vi "Keythley_2110.vi"(4 "error in":T14, 7 "Command":T15) -> (0 "error out":T14, 3 "Response":T12)   [LabVIEW 2018]
uses:
  MOKO_LabViewLibrary/MokoLowLevel/MokoLowLovelControl/MLLC_Command.ctl
  MOKO_LabViewLibrary/MokoLowLevel/MokoLowLovelControl/MLLC_Error.ctl
  MOKO_LabViewLibrary/MokoLowLevel/MokoLowLovelControl/MLLC_Mode.ctl
  MOKO_LabViewLibrary/MokoLowLevel/MokoLowLovelControl/MLLC_Response.ctl
  MOKO_LabViewLibrary/MokoLowLevel/MokoLowLovelControl/MLLC_DriverName.ctl
  MOKO_LabViewLibrary/MokoLowLevel/MokoLowLovelControl/MLLC_Request.ctl
  MOKO_LabViewLibrary/MokoLowLevel/MokoLowLovelControl/MLLC_ErrorCode.ctl
  MOKO_LabViewLibrary/MokoLowLevel/MokoLowLovelControl/MLLC_ResponseInit.ctl
  MOKO_LabViewLibrary/MokoLowLevel/MokoLowLovelControl/MLLC_ConnectCluster.ctl
  MOKO_LabViewLibrary/MokoLowLevel/MokoLowLovelControl/MLLC_InterfaceType.ctl
  MOKO_LabViewLibrary/MokoLowLevel/MokoLowLovelControl/MLLC_OpenedSession.ctl
  MOKO_LabViewLibrary/MokoLowLevel/MokoLowLovelControl/MLLC_InterfaceSettings.ctl
  MOKO_LabViewLibrary/MokoLowLevel/MokoLowLovelControl/MLLC_InterfaceKind.ctl
  data/Keythley_2110_Functions.ctl
panel:
  in  "Settings":T8={"Saved Data"=variant, "Data"={"Connect"={"InterfaceType"=enum."VISA", "OpenedSession"="USB0::0x05E6::0x2110::8000035::INSTR", "InterfaceSettings"={"Interface"=enum."USB", "EOS 4 read"=enum."LF (\\n)", "EOS 4 write"=enum."LF (\\n)", "TMO, ms"=5000, "Sett"=variant}}, "Channel"=1, "Func"=enum."VDC"}}
  in  "Response Init array":T9="KEITHLEY INSTRUMENTS INC.,MODEL 2110"
  in  "Error Code":T6=5475
  in  "Request":T10="*idn?"
  in  "Driver Name":T11="Keythley_2110"
  in  "Mode":T13=enum."Check"
  # "KEITHLEY INSTRUMENTS,MODEL DMM6500,04582450,1.7.12b = U"
  # "KEITHLEY INSTRUMENTS,MODEL DMM6500,04625545,1.7.12b = I"
  # "Keythley_2110"
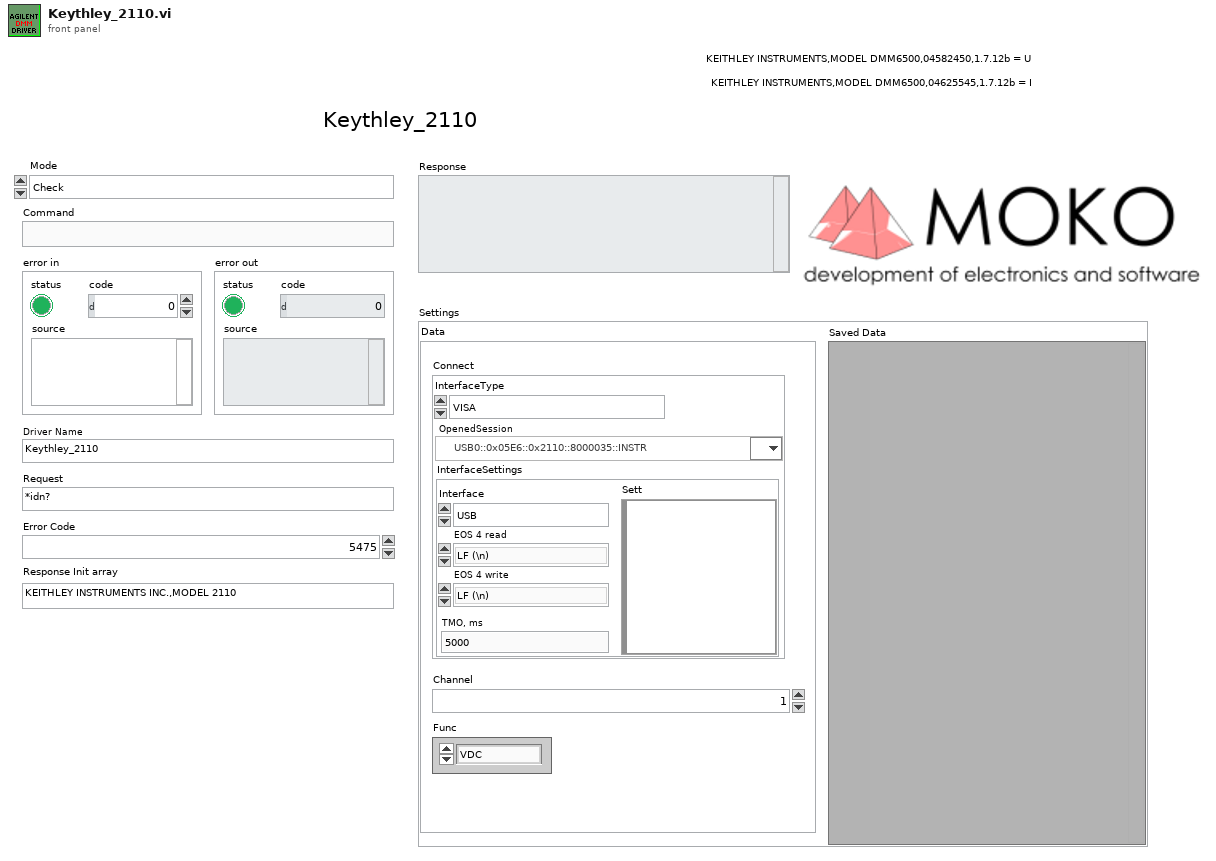
[diagram p1: front panel]
types:
  T1 = typedef "MLLC_ConnectCluster.ctl" = cluster{"InterfaceType":T2, "OpenedSession":T3, "InterfaceSettings":T4}
  T2 = typedef "MLLC_InterfaceType.ctl" = enum16{"VISA", "Prologix USB-GPIB"}
  T3 = typedef "MLLC_OpenedSession.ctl" = refnum<visa-resource-name>
  T4 = typedef "MLLC_InterfaceSettings.ctl" = cluster{"Interface":T5, "EOS 4 read":enum16{"Default (=EOS 4 write)", "CR (\\r)", "LF (\\n)", "None"}, "EOS 4 write":enum16{"CR+LF (\\r\\n)", "CR (\\r)", "LF (\\n)", "None"}, "TMO, ms":i32, "Sett":variant}
  T5 = typedef "MLLC_InterfaceKind.ctl" = enum16{"RS232", "GPIB", "USB", "Ethernet", "another"}
  T6 = typedef "MLLC_ErrorCode.ctl" = u32
  T7 = typedef "Keythley_2110_Functions.ctl" = enum16{"VDC", "VAC", "IDC", "IAC", "F", "R2", "R4", "CAP"}
  T8 = cluster{"Saved Data":variant, "Data":cluster{"Connect":T1, "Channel":T6, "Func":T7}}
  T9 = typedef "MLLC_ResponseInit.ctl" = string
  T10 = typedef "MLLC_Request.ctl" = string
  T11 = typedef "MLLC_DriverName.ctl" = string
  T12 = typedef "MLLC_Response.ctl" = string
  T13 = typedef "MLLC_Mode.ctl" = enum16{"get", "set", "close", "Init", "Check"}
  T14 = typedef "MLLC_Error.ctl" = errorcluster
  T15 = typedef "MLLC_Command.ctl" = string
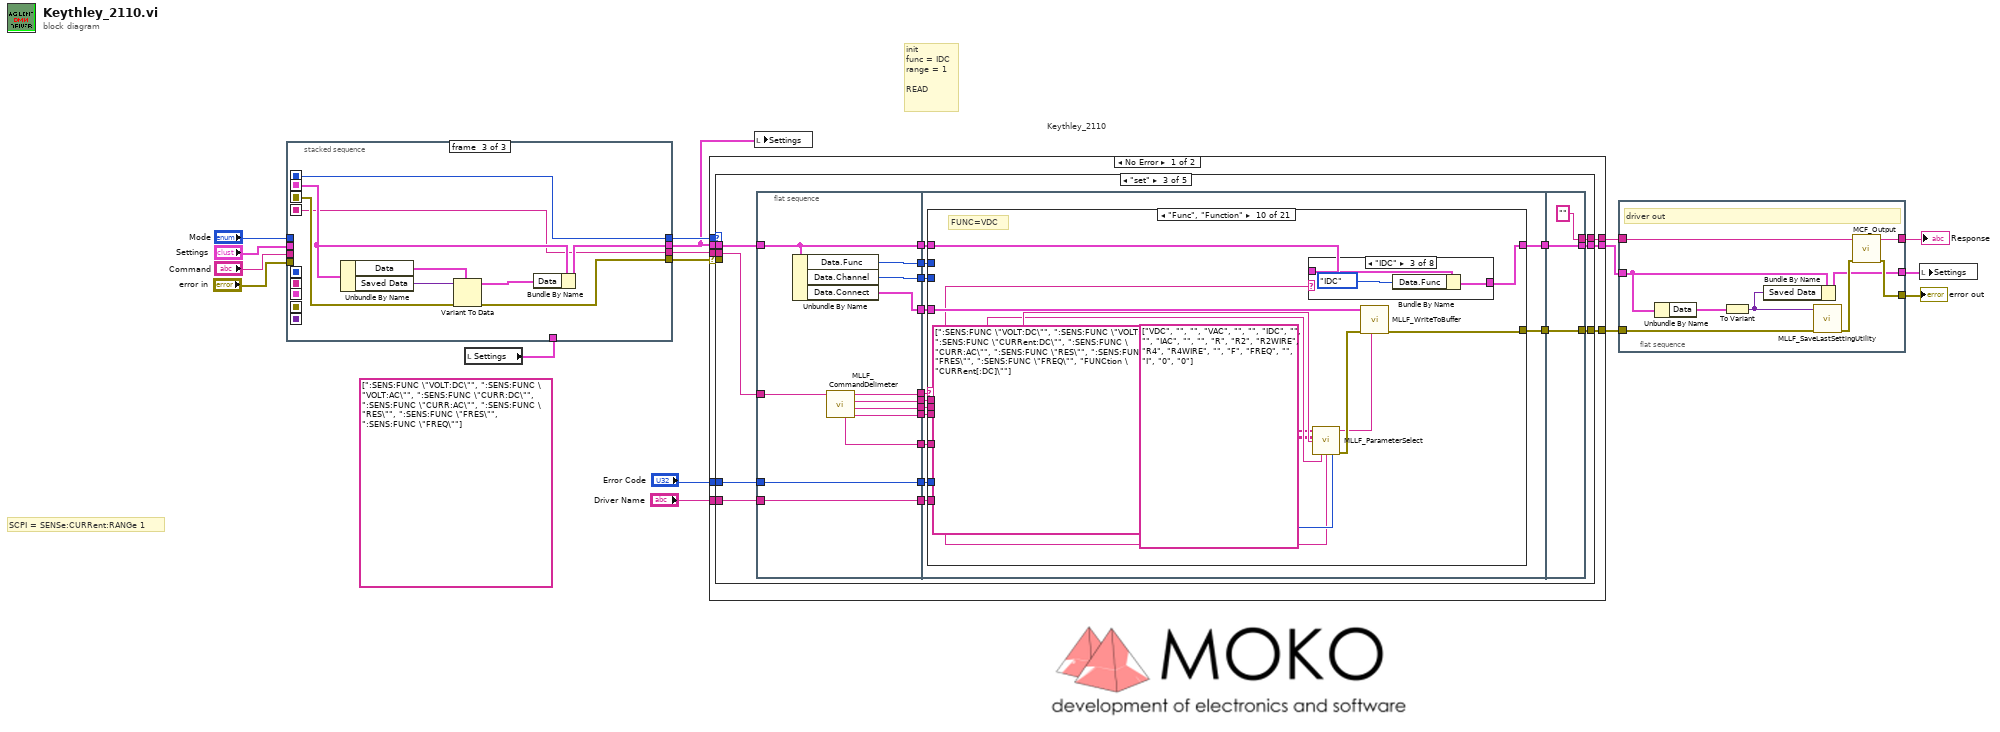
[diagram p0: block diagram]
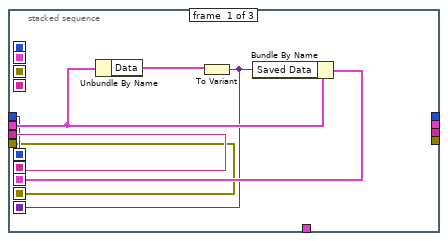
[diagram p2: hidden frame]
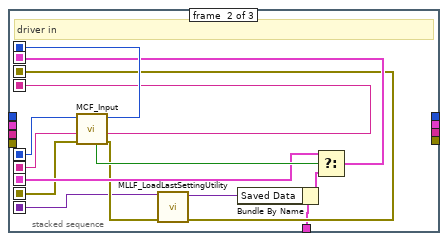
[diagram p3: hidden frame]
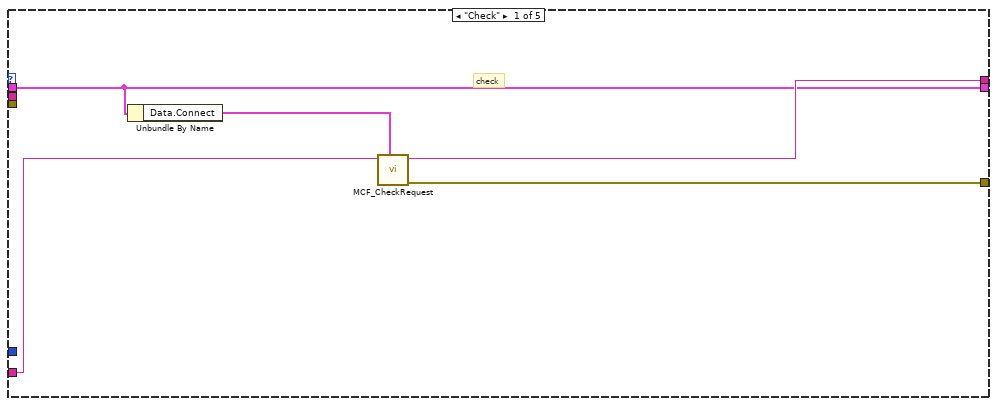
[diagram p4: hidden frame]
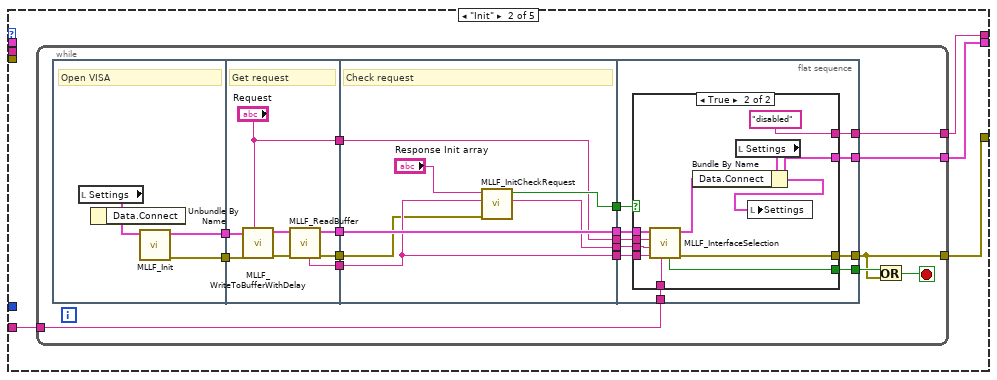
[diagram p5: hidden frame]
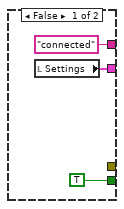
[diagram p6: hidden frame]
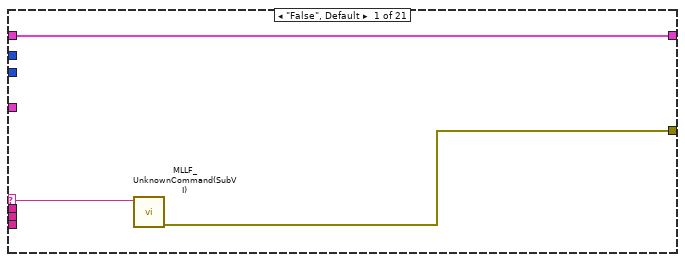
[diagram p7: hidden frame]
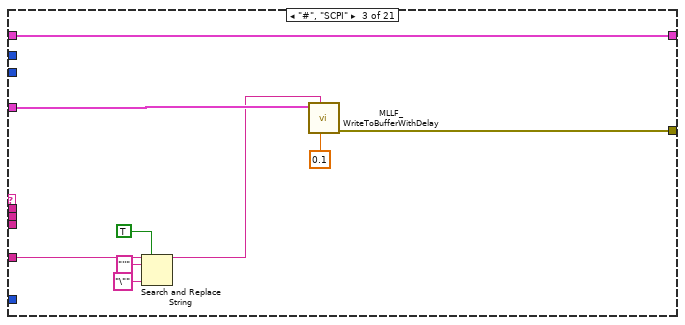
[diagram p9: hidden frame]
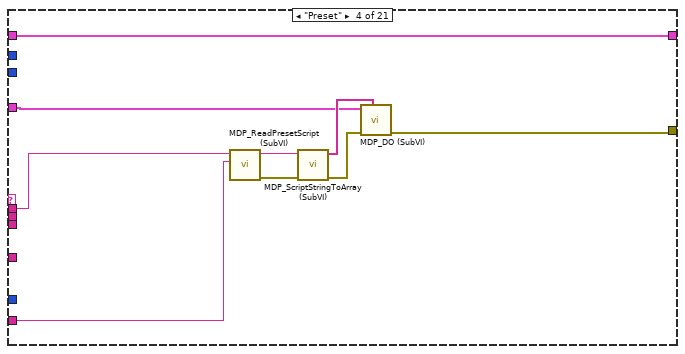
[diagram p10: hidden frame]
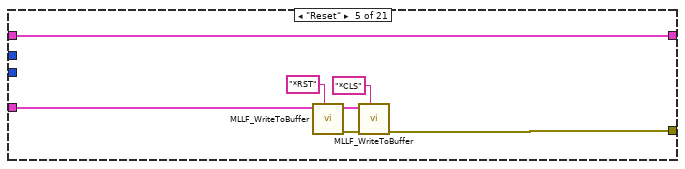
[diagram p11: hidden frame]
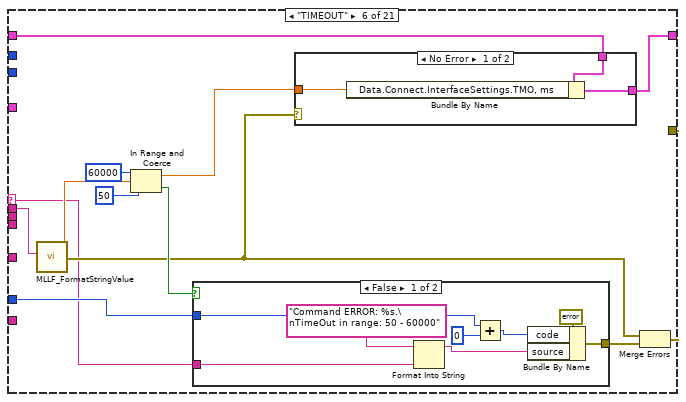
[diagram p12: hidden frame]
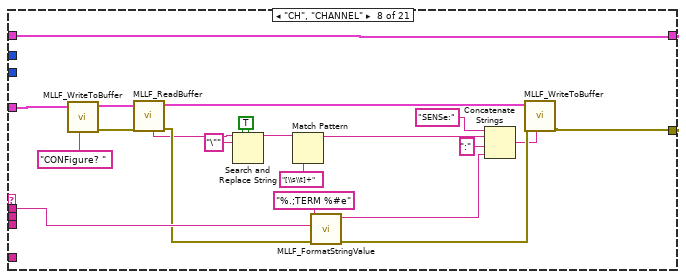
[diagram p16: hidden frame]
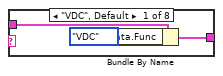
[diagram p18: hidden frame]
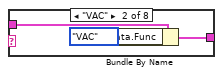
[diagram p19: hidden frame]
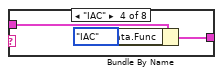
[diagram p20: hidden frame]
diagram:
  (unwired) string[] [":SENS:FUNC \"VOLT:DC\"", ":SENS:FUNC \"VOLT:AC\"", ":SENS:FUNC \"CURR:DC\"", ":SENS:FUNC \"CURR:AC\"", ":SENS:FUNC \"RES\"", ":SENS:FUNC \"FRES\"", ":SENS:FUNC \"FREQ\""] ("Names")
  # "init\nfunc = IDC\nrange = 1\n\nREAD"
  # "SCPI = SENSe:CURRent:RANGe 1"
  # "Keythley_2110"
  n1 = local read "Settings"() -> (w8:T8)
  n2 = stacked-sequence {
    seq-local: [w20 _ _] -> [_ w36 _]
    seq-local: [w19 _ _] -> [_ w37 _]
    seq-local: [w22 _ _] -> [_ w32 _]
    seq-local: [w18 _ _] -> [_ w31 _]
    seq-local: [w21 _ _] -> [_ w27 _]
    seq-local: [_ w28 _] -> [_ _ w44]
    seq-local: [_ w38 _] -> [_ _ w41]
    seq-local: [_ w35 _] -> [_ _ w40]
    seq-local: [_ w34 _] -> [_ _ w45]
    tunnel: "Command" -> [w20 _ _]
    tunnel: "Mode" -> [w19 _ _]
    tunnel: "error in" -> [w18 _ _]
    tunnel: "Settings" -> [w23 _ _]
    tunnel: w8 -> [_ w26 _]
    tunnel: [_ _ w40] -> w10
    tunnel: [_ _ w43] -> w1
    tunnel: [_ _ w42] -> w9
    tunnel: [_ _ w41] -> w11
    frame #0 {
      n3 = Unbundle By Name(w23) -> ("Data"=w24:cluster{"Connect":T1, "Channel":T6, "Func":T7})
      n4 = To Variant(anything=w24) -> (Variant=w21:variant)
      n5 = Bundle By Name(cluster=w23, "Saved Data"=w21) -> (w22:T8)
    }
    frame #1 {
      # "driver in"
      n6 = call "MCF_Input.vi"("Error In"=w31, "Command in"=w36, "Mode in"=w37) -> ("Error Out"=w30:errorcluster, "Command out"=w35:string, "Mode out"=w38:T13, "Boolean"=w33:bool)  [unwired: 5 in]
      n7 = call "MLLF_LoadLastSettingUtility.vi"("Error In"=w30, "Save data in"=w27) -> ("Error Out"=w28:errorcluster, "Save data out"=w25:variant)  [unwired: 8 in]
      n8 = Bundle By Name(cluster=w26, "Saved Data"=w25) -> (w29:T8)
      n9 = Select(t=w32, s=w33, f=w29) -> (s? t:f=w34:T8)
    }
    frame #2 {
      n10 = Unbundle By Name(w45) -> ("Data"=w46:cluster{"Connect":T1, "Channel":T6, "Func":T7}, "Saved Data"=w39:variant)
      n11 = Variant To Data(error in=w44, type=w46, Variant=w39) -> (data=w47:cluster{"Connect":T1, "Channel":T6, "Func":T7}, error out=w42:errorcluster)
      n12 = Bundle By Name(cluster=w45, "Data"=w47) -> (w43:T8)
    }
  }
  n13 = case shown="No Error" w9 {
    selector: w9 -> [w53 w615]
    tunnel: [w54 w615] -> w5
    tunnel: w11 -> [w56 _]
    tunnel: [w55 "An error occurred in the driver input module." ("String")] -> w7
    tunnel: w10 -> [w48 _]
    tunnel: w1 -> [w49 w614]
    tunnel: "Error Code" -> [w52 _]
    tunnel: "Driver Name" -> [w51 _]
    tunnel: [w50 w614] -> w6
    frame No Error {
      n14 = case shown="\"set\"" w56 {
        tunnel: [w60 w65 w139 w524 "" ("String")] -> w55
        tunnel: [w61 w63 w142 w525 w611] -> w54
        tunnel: w53 -> [_ _ _ w539 _]
        tunnel: w52 -> [_ _ w145 w541 _]
        tunnel: w51 -> [w59 w62 w143 w540 _]
        tunnel: [w58 w64 w144 w542 w610] -> w50
        tunnel: w49 -> [w58 _ w128 w530 w610]
        tunnel: w48 -> [_ _ w127 w529 _]
        frame "Check" {
          # "check"
          n15 = Unbundle By Name(w58) -> ("Data.Connect"=w57:T1)
          n16 = call "MCF_CheckRequest.vi"("Permanent data.Connect"=w57, "Driver Name"=w59) -> ("Error Out"=w61:errorcluster, "Output String"=w60:string)  [unwired: 8 in]
        }
        frame "Init" {
          n17 = while {
            tunnel: [w71] -> w63
            tunnel: [w70] -> w65
            tunnel: [w69] -> w64
            tunnel: w62 -> [w73]
            stop <- w82 stop-if-true
            n18 = flat-sequence {
              tunnel: [w86] -> w81
              tunnel: [w85] -> w80
              tunnel: w81 -> [w92]
              tunnel: w80 -> [w91]
              tunnel: [w90] -> w79
              tunnel: [w89] -> w78
              tunnel: [w88] -> w77
              tunnel: ["Request"] -> w67
              tunnel: w79 -> [w98]
              tunnel: w78 -> [w101]
              tunnel: w77 -> [w100]
              tunnel: [w101] -> w76
              tunnel: [w100] -> w75
              tunnel: [w97] -> w74
              tunnel: [w96] -> w68
              tunnel: w67 -> [w95]
              tunnel: [w95] -> w66
              tunnel: w76 -> [w110]
              tunnel: w75 -> [w109]
              tunnel: w74 -> [w111]
              tunnel: w73 -> [w108]
              tunnel: [w107] -> w72
              tunnel: [w106] -> w71
              tunnel: [w105] -> w70
              tunnel: [w104] -> w69
              tunnel: w68 -> [w103]
              tunnel: w66 -> [w102]
              frame #0 {
                # "Open VISA"
                n19 = local read "Settings"() -> (w84:T8)
                n20 = Unbundle By Name(w84) -> ("Data.Connect"=w83:T1)
                n21 = call "MLLF_Init.vi"("DriverConnect in"=w83) -> ("Error Out"=w86:errorcluster, "DriverConnect out"=w85:T1)  [unwired: 7 in]
              }
              frame #1 {
                # "Get request"
                n22 = call "MLLF_WriteToBufferWithDelay.vi"("Command"="Request", "Error In"=w92, "DriverConnect in"=w91) -> ("Error Out"=w93:errorcluster, "DriverConnect out"=w94:T1)  [unwired: 7 in]
                n23 = call "MLLF_ReadBuffer.vi"("Error In"=w93, "DriverConnect in"=w94) -> ("Error Out"=w90:errorcluster, "DriverConnect out"=w89:T1, "String"=w88:string)  [unwired: 6 in]
              }
              frame #2 {
                # "Check request"
                n24 = call "MLLF_InitCheckRequest.vi"("error in (no error)"=w98, "Answer"=w100, "Response Init"="Response Init array") -> ("ResponseInit out"=w96:string, "Design"=w97:bool)  [unwired: 5 in, 2 out]
              }
              frame #3 {
                n25 = case shown="True" w111 {
                  tunnel: w110 -> [_ w124]
                  tunnel: [TRUE w119] -> w107
                  tunnel: [_ w122] -> w106
                  tunnel: ["connected" "disabled"] -> w105
                  tunnel: [w112 w120] -> w104
                  tunnel: w109 -> [_ w117]
                  tunnel: w108 -> [_ w118]
                  tunnel: w103 -> [_ w116]
                  tunnel: w102 -> [_ w115]
                  frame False {
                    n26 = local read "Settings"() -> (w112:T8)
                  }
                  frame True {
                    n27 = call "MLLF_InterfaceSelection.vi"("Driver Name"=w118, "Answer:"=w117, "Response"=w116, "Request"=w115, "DriverConnect in"=w124) -> ("error out"=w122:T14, "DriverConnect out"=w123:T1, "stop init?"=w119:bool)  [unwired: 2 in, 2 out]
                    n28 = local read "Settings"() -> (w125:T8)
                    n29 = Bundle By Name(cluster=w125, "Data.Connect"=w123) -> (w120:T8)
                    n30 = local write "Settings"(w120) -> ()
                  }
                }
              }
            }
            n31 = Or(x=w72, y=w71) -> (x .or. y?=w82:bool)
          }
        }
        frame "set" {
          n32 = flat-sequence {
            tunnel: w143 -> [w156]
            tunnel: w128 -> [w147]
            tunnel: w145 -> [w157]
            tunnel: [w157] -> w138
            tunnel: [w147] -> w137
            tunnel: [w156] -> w136
            tunnel: [w153] -> w135
            tunnel: [w154] -> w134
            tunnel: [w155] -> w133
            tunnel: [w148] -> w132
            tunnel: [w149] -> w131
            tunnel: [w150] -> w130
            tunnel: [w151] -> w129
            tunnel: w127 -> [w152]
            tunnel: [w146] -> w126
            tunnel: [w168] -> w141
            tunnel: [w161] -> w140
            tunnel: w138 -> [w170]
            tunnel: w137 -> [w169]
            tunnel: w136 -> [w167]
            tunnel: w135 -> [w166]
            tunnel: w134 -> [w165]
            tunnel: w133 -> [w164]
            tunnel: w132 -> [w163]
            tunnel: w131 -> [w162]
            tunnel: w130 -> [w160]
            tunnel: w129 -> [w159]
            tunnel: w126 -> [w158]
            tunnel: [w522] -> w142
            tunnel: [w523] -> w144
            tunnel: w141 -> [w523]
            tunnel: w140 -> [w522]
            tunnel: ["" ("String")] -> w139
            frame #0 {
              n33 = Unbundle By Name(w147) -> ("Data.Func"=w155:T7, "Data.Channel"=w154:T6, "Data.Connect"=w153:T1)
              n34 = call "MLLF_CommandDelimeter.vi"("command with param"=w152) -> ("param 3"=w151:string, "param 2"=w150:string, "param 1"=w149:string, "command"=w148:string, "Spit delimetre"=w146:string)  [unwired: 6 in]
            }
            frame #1 {
              n35 = case shown="\"Func\", \"Function\"" w163 {
                selector: w163 -> [w172 _ _ _ _ w201 _ _ _ w253 _ _ _ _ _ _ w445 w452 w476 w500 w511]
                tunnel: w162 -> [_ _ _ w187 _ w200 _ w244 _ w254 w293 _ w323 w336 w377 w407 w446 w453 w477 w501 w512]
                tunnel: [w171 _ w180 w184 w193 w206 _ w226 _ w248 w288 _ w306 w335 w361 w392 w425 w451 w475 w499 w510] -> w161
                tunnel: w170 -> [_ _ _ _ _ w207 _ _ _ w259 _ _ _ _ _ _ w447 w457 w481 w505 w519]
                tunnel: w169 -> [w173 w174 w183 w192 w199 w211 w225 w245 w247 w256 w294 w305 w325 w352 w379 w409 w450 w474 w498 w509 w520]
                tunnel: [w173 w174 w183 w192 w199 w212 w225 w245 w247 w255 w294 w305 w325 w352 w379 w409 w450 w474 w498 w509 w520] -> w168
                tunnel: w166 -> [_ _ w181 w185 w194 _ _ w246 _ w257 w286 _ w324 w351 w378 w408 w449 w473 w497 w503 w516]
                tunnel: w167 -> [_ _ _ w186 _ _ _ _ _ w258 _ _ _ _ _ _ w448 w458 w482 w506 w518]
                tunnel: w165 -> [_ _ _ _ _ _ _ _ _ _ _ _ _ _ _ _ _ _ _ _ _]
                tunnel: w164 -> [_ _ _ _ _ _ _ _ _ _ w287 _ _ _ _ _ _ _ _ _ _]
                tunnel: w160 -> [_ _ _ _ _ _ _ _ _ _ _ _ _ _ _ _ _ _ _ _ _]
                tunnel: w159 -> [_ _ _ _ _ _ _ _ _ _ _ _ _ _ _ _ _ _ _ _ _]
                tunnel: w158 -> [_ _ w179 _ _ _ _ _ _ _ _ _ _ _ _ _ _ _ _ _ _]
                frame "False", Default {
                  n36 = call "MLLF_UnknownCommand(SubVI).vi"("Unknown command"=w172) -> ("error out"=w171:errorcluster)  [unwired: 10 in]
                }
                frame "______________ Standart ________________" {
                }
                frame "#", "SCPI" {
                  n37 = Search and Replace String(replace all?=TRUE ("replace all? (F)"), input string=w179, search string="''", replace string="\"" ("replace string (\"\")")) -> (result string=w175:string)  [unwired: 4 in, 3 out]
                  n38 = call "MLLF_WriteToBufferWithDelay.vi"("Delay Time ( 0,05 s)"=0.1 ("Delay Time (s)"), "Command"=w175, "DriverConnect in"=w181) -> ("Error Out"=w180:errorcluster)  [unwired: 7 in, 1 out]
                }
                frame "Preset" {
                  n39 = call "MDP_ReadPresetScript (SubVI).vi"("Driver Name"=w186, "String in"=w187) -> ("Error Out"=w189:errorcluster, "String out"=w190:string)  [unwired: 8 in]
                  n40 = call "MDP_ScriptStringToArray (SubVI).vi"("Error In"=w189, "String script"=w190) -> ("Error Out"=w191:errorcluster, "Array script"=w188:string[])  [unwired: 8 in]
                  n41 = call "MDP_DO (SubVI).vi"("Array script"=w188, "Error in (no error)"=w191, "DriverConnect in"=w185) -> ("Error Out"=w184:errorcluster)  [unwired: 7 in, 1 out]
                }
                frame "Reset" {
                  n42 = call "MLLF_WriteToBuffer.vi"("String"="*RST", "DriverConnect in"=w194) -> ("error out"=w197:T14, "DriverConnect out"=w198:T1)  [unwired: 6 in]
                  n43 = call "MLLF_WriteToBuffer.vi"("String"="*CLS" ("write buffer"), "error in"=w197, "DriverConnect in"=w198) -> ("error out"=w193:T14)  [unwired: 5 in, 1 out]
                }
                frame "TIMEOUT" {
                  n44 = call "MLLF_FormatStringValue.vi"("String Value"=w200) -> ("error out"=w202:T14, "number"=w203:dbl)  [unwired: 8 in, 1 out]
                  n45 = In Range and Coerce(upper limit=60000, x=w203, lower limit=50) -> (coerced(x)=w208:dbl, In Range?=w204:bool)
                  n46 = case shown="False" w204 {
                    tunnel: [w219 _] -> w205
                    tunnel: w207 -> [w218 _]
                    tunnel: w201 -> [w217 _]
                    frame False {
                      n47 = Format Into String(format string="Command ERROR: %s.\nTimeOut in range: 50 - 60000", w217) -> (resulting string=w221:string)  [unwired: 2 in, 1 out]
                      n48 = Add(x=w218, y=0) -> (x+y=w222:T6)
                      n49 = Bundle By Name(cluster=errorcluster {"status"=TRUE, "code"=0, "source"=""} ("error out"), "code"=w222, "source"=w221) -> (w219:errorcluster)
                    }
                    frame True {
                    }
                  }
                  n50 = case shown="No Error" w202 {
                    tunnel: [w215 w216] -> w212
                    tunnel: w211 -> [w214 w216]
                    tunnel: w208 -> [w213 _]
                    frame No Error {
                      n51 = Bundle By Name(cluster=w214, "Data.Connect.InterfaceSettings.TMO, ms"=w213) -> (w215:T8)
                    }
                    frame Error {
                    }
                  }
                  n52 = Merge Errors(w202, w205) -> (w206:errorcluster)
                }
                frame "________________________________________" {
                }
                frame "CH", "CHANNEL" {
                  w231 = TRUE ("replace all? (F)")
                  n53 = call "MLLF_WriteToBuffer.vi"("String"="CONFigure? ", "DriverConnect in"=w246) -> ("error out"=w240:T14, "DriverConnect out"=w241:T1)  [unwired: 6 in]
                  n54 = call "MLLF_ReadBuffer.vi"("Error In"=w240, "DriverConnect in"=w241) -> ("Error Out"=w239:errorcluster, "DriverConnect out"=w238:T1, "String"=w233:string)  [unwired: 6 in]
                  n55 = Search and Replace String(replace all?=w231, case sensitive?=w231, input string=w233, search string="\"") -> (result string=w232:string)  [unwired: 4 in, 3 out]
                  n56 = Match Pattern(string=w232, regular expression="[\\s\\t]+") -> (before substring=w234:string)  [unwired: 1 in, 3 out]
                  n57 = call "MLLF_FormatStringValue.vi"("error in"=w239, "String Value"=w244, "Format"="%.;TERM %#e" ("format string")) -> ("error out"=w243:T14, "String Value Formated"=w236:T15)  [unwired: 6 in, 1 out]
                  n58 = Concatenate Strings("SENSe:" ("string"), w234, ":" ("string"), w236) -> (w229:string)
                  n59 = call "MLLF_WriteToBuffer.vi"("String"=w229, "error in"=w243, "DriverConnect in"=w238) -> ("error out"=w226:T14)  [unwired: 5 in, 1 out]
                }
                frame "<----MAIN FUNCTIONS---->" {
                }
                frame "Func", "Function" {
                  # "FUNC=VDC"
                  n60 = case shown="\"IDC\"" w254 {
                    tunnel: w256 -> [w262 w265 w268 w271 w274 w277 w280 w283]
                    tunnel: [w261 w264 w267 w270 w273 w276 w279 w282] -> w255
                    frame "VDC", Default {
                      n61 = Bundle By Name(cluster=w262, "Data.Func"=Keythley_2110_Functions."VDC" ("Func")) -> (w261:T8)
                    }
                    frame "VAC" {
                      n62 = Bundle By Name(cluster=w265, "Data.Func"=Keythley_2110_Functions."VAC" ("Func")) -> (w264:T8)
                    }
                    frame "IDC" {
                      n63 = Bundle By Name(cluster=w268, "Data.Func"=Keythley_2110_Functions."IDC" ("Func")) -> (w267:T8)
                    }
                    frame "IAC" {
                      n64 = Bundle By Name(cluster=w271, "Data.Func"=Keythley_2110_Functions."IAC" ("Func")) -> (w270:T8)
                    }
                    frame "R", "R2", "R2WI" {
                      n65 = Bundle By Name(cluster=w274, "Data.Func"=Keythley_2110_Functions."R2" ("Func")) -> (w273:T8)
                    }
                    frame "R4", "R4WI" {
                      n66 = Bundle By Name(cluster=w277, "Data.Func"=Keythley_2110_Functions."R4" ("Func")) -> (w276:T8)
                    }
                    frame "F" {
                      n67 = Bundle By Name(cluster=w280, "Data.Func"=Keythley_2110_Functions."F" ("Func")) -> (w279:T8)
                    }
                    frame "C", "CAP" {
                      n68 = Bundle By Name(cluster=w283, "Data.Func"=Keythley_2110_Functions."CAP" ("Func")) -> (w282:T8)
                    }
                  }
                  n69 = call "MLLF_ParameterSelect.vi"("Command to equipment"=string[] [":SENS:FUNC \"VOLT:DC\"", ":SENS:FUNC \"VOLT:AC\"", ":SENS:FUNC \"CURRent:DC\"", ":SENS:FUNC \"CURR:AC\"", ":SENS:FUNC \"RES\"", ":SENS:FUNC \"FRES\"", ":SENS:FUNC \"FREQ\"", "FUNCtion \"CURRent[:DC]\""] ("Names"), "Names"=string[][] [["VDC", "", ""], ["VAC", "", ""], ["IDC", "", ""], ["IAC", "", ""], ["R", "R2", "R2WIRE"], ["R4", "R4WIRE", ""], ["F", "FREQ", ""], ["I", "0", "0"]], "Input"=w254, "Command"=w253, "Driver Name"=w258, "Error Code"=w259) -> ("Choice"=w249:string, "Error Out"=w250:errorcluster)  [unwired: 8 in]
                  n70 = call "MLLF_WriteToBuffer.vi"("String"=w249, "error in"=w250, "DriverConnect in"=w257) -> ("error out"=w248:T14)  [unwired: 5 in, 1 out]
                }
                frame "Range" {
                  n71 = case shown="\"IDC\"" w287 {
                    tunnel: ["VOLT" ("String") "VOLT:AC" ("String") "CURR:DC" ("String")] -> w285
                    frame "VDC", Default {
                    }
                    frame "VAC" {
                    }
                    frame "IDC" {
                    }
                  }
                  n72 = case shown="Default" w293 {
                    selector: w293 -> [w298 _ _ _]
                    tunnel: [w301 _ _ _] -> w292
                    tunnel: [w300 "RANG:AUTO ON" ("String") "RANG MIN" ("String") "RANG MAX" ("String")] -> w291
                    frame Default {
                      n73 = call "MLLF_FormatStringValue.vi"("String Value"=w298, "Format"="RANG %#e" ("format string")) -> ("error out"=w301:T14, "String Value Formated"=w300:T15)  [unwired: 7 in, 1 out]
                    }
                    frame "Auto" {
                    }
                    frame "MIN" {
                    }
                    frame "MAX" {
                    }
                  }
                  n74 = Concatenate Strings("SENSe:" ("string"), w285, ":" ("string"), w291) -> (w289:string)
                  n75 = call "MLLF_WriteToBuffer.vi"("String"=w289, "error in"=w292, "DriverConnect in"=w286) -> ("error out"=w288:T14)  [unwired: 5 in, 1 out]
                }
                frame "---------ADDITIONAL---------" {
                }
                frame "Res", "Resolution" {
                  w310 = TRUE ("replace all? (F)")
                  n76 = call "MLLF_WriteToBuffer.vi"("String"="CONFigure? ", "DriverConnect in"=w324) -> ("error out"=w319:T14, "DriverConnect out"=w320:T1)  [unwired: 6 in]
                  n77 = call "MLLF_ReadBuffer.vi"("Error In"=w319, "DriverConnect in"=w320) -> ("Error Out"=w318:errorcluster, "DriverConnect out"=w317:T1, "String"=w312:string)  [unwired: 6 in]
                  n78 = Search and Replace String(replace all?=w310, case sensitive?=w310, input string=w312, search string="\"") -> (result string=w311:string)  [unwired: 4 in, 3 out]
                  n79 = case shown="\"MIN\"" w323 {
                    selector: w323 -> [w327 _ _]
                    tunnel: [w330 w331 w333] -> w322
                    tunnel: [w329 "RES MAX" ("String") "RES MIN" ("String")] -> w315
                    tunnel: w318 -> [w326 w331 w333]
                    frame "False", Default {
                      n80 = call "MLLF_FormatStringValue.vi"("error in"=w326, "String Value"=w327, "Format"="RES %#e" ("format string")) -> ("error out"=w330:T14, "String Value Formated"=w329:T15)  [unwired: 6 in, 1 out]
                    }
                    frame "MAX" {
                    }
                    frame "MIN" {
                    }
                  }
                  n81 = Match Pattern(string=w311, regular expression="[\\s\\t]+") -> (before substring=w313:string)  [unwired: 1 in, 3 out]
                  n82 = Concatenate Strings("SENSe:" ("string"), w313, ":" ("string"), w315) -> (w308:string)
                  n83 = call "MLLF_WriteToBuffer.vi"("String"=w308, "error in"=w322, "DriverConnect in"=w317) -> ("error out"=w306:T14)  [unwired: 5 in, 1 out]
                }
                frame "Aper", "Aperture", "MeasTime" {
                  w339 = TRUE ("replace all? (F)")
                  n84 = call "MLLF_WriteToBuffer.vi"("String"="CONFigure? ", "DriverConnect in"=w351) -> ("error out"=w348:T14, "DriverConnect out"=w349:T1)  [unwired: 6 in]
                  n85 = call "MLLF_ReadBuffer.vi"("Error In"=w348, "DriverConnect in"=w349) -> ("Error Out"=w347:errorcluster, "DriverConnect out"=w346:T1, "String"=w341:string)  [unwired: 6 in]
                  n86 = Search and Replace String(replace all?=w339, case sensitive?=w339, input string=w341, search string="\"") -> (result string=w340:string)  [unwired: 4 in, 3 out]
                  n87 = case shown="\"OFF\"" w336 {
                    selector: w336 -> [w355 _]
                    tunnel: [w358 w359] -> w353
                    tunnel: [w357 "APER:ENAB OFF" ("String")] -> w344
                    tunnel: w347 -> [w354 w359]
                    frame "False", Default {
                      n88 = call "MLLF_FormatStringValue.vi"("error in"=w354, "String Value"=w355, "Format"="APER %#e" ("format string")) -> ("error out"=w358:T14, "String Value Formated"=w357:T15)  [unwired: 6 in, 1 out]
                    }
                    frame "OFF" {
                    }
                  }
                  n89 = Match Pattern(string=w340, regular expression="[\\s\\t]+") -> (before substring=w342:string)  [unwired: 1 in, 3 out]
                  n90 = Concatenate Strings(w342, ":" ("string"), w344) -> (w337:string)
                  n91 = call "MLLF_WriteToBuffer.vi"("String"=w337, "error in"=w353, "DriverConnect in"=w346) -> ("error out"=w335:T14)  [unwired: 5 in, 1 out]
                }
                frame "IntegrationTime", "IntTime", "NPLC" {
                  w365 = TRUE ("replace all? (F)")
                  n92 = call "MLLF_WriteToBuffer.vi"("String"="CONFigure? ", "DriverConnect in"=w378) -> ("error out"=w373:T14, "DriverConnect out"=w374:T1)  [unwired: 6 in]
                  n93 = call "MLLF_ReadBuffer.vi"("Error In"=w373, "DriverConnect in"=w374) -> ("DriverConnect out"=w372:T1, "String"=w367:string)  [unwired: 6 in, 1 out]
                  n94 = Search and Replace String(replace all?=w365, case sensitive?=w365, input string=w367, search string="\"") -> (result string=w366:string)  [unwired: 4 in, 3 out]
                  n95 = case shown="\"MIN\"" w377 {
                    tunnel: [w383 w387 w391] -> w376
                    tunnel: [w382 w386 w390] -> w370
                    tunnel: w377 -> [w380 w384 w388]
                    frame Default {
                      n96 = call "MLLF_FormatStringValue.vi"("String Value"=w380, "Format"="NPLC %#e" ("format string")) -> ("error out"=w383:T14, "String Value Formated"=w382:T15)  [unwired: 7 in, 1 out]
                    }
                    frame "MIN" {
                      n97 = call "MLLF_FormatStringValue.vi"("String Value"=w384, "Format"="NPLC MIN" ("format string")) -> ("error out"=w387:T14, "String Value Formated"=w386:T15)  [unwired: 7 in, 1 out]
                    }
                    frame "MAX" {
                      n98 = call "MLLF_FormatStringValue.vi"("String Value"=w388, "Format"="NPLC MAX" ("format string")) -> ("error out"=w391:T14, "String Value Formated"=w390:T15)  [unwired: 7 in, 1 out]
                    }
                  }
                  n99 = Match Pattern(string=w366, regular expression="[\\s\\t]+") -> (before substring=w368:string)  [unwired: 1 in, 3 out]
                  n100 = Concatenate Strings("SENSe:" ("string"), w368, ":" ("string"), w370) -> (w363:string)
                  n101 = call "MLLF_WriteToBuffer.vi"("String"=w363, "error in"=w376, "DriverConnect in"=w372) -> ("error out"=w361:T14)  [unwired: 5 in, 1 out]
                }
                frame "ACBand", "ACBandwidth", "Band", "Bandwidth" {
                  w396 = TRUE ("replace all? (F)")
                  n102 = call "MLLF_WriteToBuffer.vi"("String"="CONFigure? ", "DriverConnect in"=w408) -> ("error out"=w403:T14, "DriverConnect out"=w404:T1)  [unwired: 6 in]
                  n103 = call "MLLF_ReadBuffer.vi"("Error In"=w403, "DriverConnect in"=w404) -> ("Error Out"=w402:errorcluster, "DriverConnect out"=w401:T1, "String"=w398:string)  [unwired: 6 in]
                  n104 = case shown="\"MAX\"" w407 {
                    tunnel: [w414 w419 w424] -> w406
                    tunnel: w402 -> [w413 w418 w423]
                    tunnel: [w412 w417 w422] -> w399
                    tunnel: w407 -> [w410 w415 w420]
                    frame Default {
                      n105 = call "MLLF_FormatStringValue.vi"("error in"=w413, "String Value"=w410, "Format"="BAND %#f" ("format string")) -> ("error out"=w414:T14, "String Value Formated"=w412:T15)  [unwired: 6 in, 1 out]
                    }
                    frame "MAX" {
                      n106 = call "MLLF_FormatStringValue.vi"("error in"=w418, "String Value"=w415, "Format"="BAND MAX" ("format string")) -> ("error out"=w419:T14, "String Value Formated"=w417:T15)  [unwired: 6 in, 1 out]
                    }
                    frame "MIN" {
                      n107 = call "MLLF_FormatStringValue.vi"("error in"=w423, "String Value"=w420, "Format"="BAND MIN" ("format string")) -> ("error out"=w424:T14, "String Value Formated"=w422:T15)  [unwired: 6 in, 1 out]
                    }
                  }
                  n108 = Search and Replace String(replace all?=w396, case sensitive?=w396, input string=w398, search string="\"") -> (result string=w397:string)  [unwired: 4 in, 3 out]
                  n109 = Match Pattern(string=w397, regular expression="[\\s\\t]+") -> ()  [unwired: 1 in, 4 out]
                  n110 = Concatenate Strings(":DET:" ("string"), w399) -> (w394:string)
                  n111 = call "MLLF_WriteToBuffer.vi"("String"=w394, "error in"=w406, "DriverConnect in"=w401) -> ("error out"=w392:T14)  [unwired: 5 in, 1 out]
                }
                frame "AutoZero", "ZERO" {
                  w435 = TRUE ("replace all? (F)")
                  n112 = call "MLLF_WriteToBuffer.vi"("String"="CONFigure? ", "DriverConnect in"=w449) -> ("error out"=w442:T14, "DriverConnect out"=w443:T1)  [unwired: 6 in]
                  n113 = call "MLLF_ReadBuffer.vi"("Error In"=w442, "DriverConnect in"=w443) -> ("Error Out"=w429:errorcluster, "DriverConnect out"=w441:T1, "String"=w437:string)  [unwired: 6 in]
                  n114 = Search and Replace String(replace all?=w435, case sensitive?=w435, input string=w437, search string="\"") -> (result string=w436:string)  [unwired: 4 in, 3 out]
                  n115 = Match Pattern(string=w436, regular expression="[\\s\\t]+") -> (before substring=w438:string)  [unwired: 1 in, 3 out]
                  n116 = call "MLLF_ParameterSelect.vi"("Command to equipment"=string[] ["ZERO:AUTO OFF", "ZERO:AUTO ON", "ZERO:AUTO ONCE"] ("Names"), "Ignor case(default = true)"=TRUE, "Names"=string[][] [["OFF"], ["ON"], ["ONCE"]], "Input"=w446, "Error In"=w429, "Command"=w445, "Driver Name"=w448, "Error Code"=w447) -> ("Choice"=w428:string, "Error Out"=w430:errorcluster)  [unwired: 6 in]
                  n117 = Concatenate Strings("SENSe:" ("string"), w438, ":" ("string"), w428) -> (w433:string)
                  n118 = call "MLLF_WriteToBuffer.vi"("String"=w433, "error in"=w430, "DriverConnect in"=w441) -> ("error out"=w425:T14)  [unwired: 5 in, 1 out]
                }
                frame "LOWPOWER" {
                  w463 = TRUE ("replace all? (F)")
                  n119 = call "MLLF_WriteToBuffer.vi"("String"="CONFigure? ", "DriverConnect in"=w473) -> ("error out"=w470:T14, "DriverConnect out"=w471:T1)  [unwired: 6 in]
                  n120 = call "MLLF_ReadBuffer.vi"("Error In"=w470, "DriverConnect in"=w471) -> ("Error Out"=w455:errorcluster, "DriverConnect out"=w469:T1, "String"=w465:string)  [unwired: 6 in]
                  n121 = Search and Replace String(replace all?=w463, case sensitive?=w463, input string=w465, search string="\"") -> (result string=w464:string)  [unwired: 4 in, 3 out]
                  n122 = Match Pattern(string=w464, regular expression="[\\s\\t]+") -> (before substring=w466:string)  [unwired: 1 in, 3 out]
                  n123 = call "MLLF_ParameterSelect.vi"("Command to equipment"=string[] ["POW:LIM OFF", "POW:LIM ON"] ("Names"), "Names"=string[][] [["0", "DIS", "DISABLE", "DISABLED", "OFF"], ["1", "EN", "ENABLE", "ENABLED", "ON"]], "Input"=w453, "Error In"=w455, "Command"=w452, "Driver Name"=w458, "Error Code"=w457) -> ("Choice"=w454:string, "Error Out"=w456:errorcluster)  [unwired: 7 in]
                  n124 = Concatenate Strings(w466, ":" ("string"), w454) -> (w461:string)
                  n125 = call "MLLF_WriteToBuffer.vi"("String"=w461, "error in"=w456, "DriverConnect in"=w469) -> ("error out"=w451:T14)  [unwired: 5 in, 1 out]
                }
                frame "VOLTAGELIMITED" {
                  w487 = TRUE ("replace all? (F)")
                  n126 = call "MLLF_WriteToBuffer.vi"("String"="CONFigure? ", "DriverConnect in"=w497) -> ("error out"=w494:T14, "DriverConnect out"=w495:T1)  [unwired: 6 in]
                  n127 = call "MLLF_ReadBuffer.vi"("Error In"=w494, "DriverConnect in"=w495) -> ("Error Out"=w479:errorcluster, "DriverConnect out"=w493:T1, "String"=w489:string)  [unwired: 6 in]
                  n128 = Search and Replace String(replace all?=w487, case sensitive?=w487, input string=w489, search string="\"") -> (result string=w488:string)  [unwired: 4 in, 3 out]
                  n129 = Match Pattern(string=w488, regular expression="[\\s\\t]+") -> (before substring=w490:string)  [unwired: 1 in, 3 out]
                  n130 = call "MLLF_ParameterSelect.vi"("Command to equipment"=string[] ["VOLT:LIM OFF", "VOLT:LIM ON"] ("Names"), "Names"=string[][] [["0", "DIS", "DISABLE", "DISABLED", "OFF"], ["1", "EN", "ENABLE", "ENABLED", "ON"]], "Input"=w477, "Error In"=w479, "Command"=w476, "Driver Name"=w482, "Error Code"=w481) -> ("Choice"=w478:string, "Error Out"=w480:errorcluster)  [unwired: 7 in]
                  n131 = Concatenate Strings(w490, ":" ("string"), w478) -> (w485:string)
                  n132 = call "MLLF_WriteToBuffer.vi"("String"=w485, "error in"=w480, "DriverConnect in"=w493) -> ("error out"=w475:T14)  [unwired: 5 in, 1 out]
                }
                frame "FILT", "FILTER" {
                  # "FILT=DIS"
                  n133 = call "MLLF_ParameterSelect.vi"("Command to equipment"=string[] ["INPut:FILTer:STATE OFF", "INPut:FILTer:STATE ON"] ("Names"), "Names"=string[][] [["0", "DIS", "DISABLE", "DISABLED", "OFF"], ["1", "EN", "ENABLE", "ENABLED", "ON"]], "Input"=w501, "Command"=w500, "Driver Name"=w506, "Error Code"=w505) -> ("Choice"=w502:string, "Error Out"=w504:errorcluster)  [unwired: 8 in]
                  n134 = call "MLLF_WriteToBuffer.vi"("String"=w502, "error in"=w504, "DriverConnect in"=w503) -> ("error out"=w499:T14)  [unwired: 5 in, 1 out]
                }
                frame "SND", "Sound" {
                  # "sound"
                  # "sound=off"
                  n135 = call "MLLF_ParameterSelect.vi"("Command to equipment"=string[] ["SYST:BEEP:STAT OFF", "SYST:BEEP:STAT ON", "SYST:BEEP"] ("Names"), "Names"=string[][] [["0", "DIS", "DISABLED", "DISABLE", "OFF"], ["1", "EN", "ENABLE", "ENABLED", "ON"], [" ", "", "", "", ""]], "Input"=w512, "Command"=w511, "Driver Name"=w518, "Error Code"=w519) -> ("Choice"=w515:string, "Error Out"=w517:errorcluster)  [unwired: 8 in]
                  n136 = call "MLLF_WriteToBuffer.vi"("String"=w515, "error in"=w517, "DriverConnect in"=w516) -> ("error out"=w510:T14)  [unwired: 5 in, 1 out]
                }
              }
            }
            frame #2 {
            }
          }
        }
        frame "get" {
          n137 = flat-sequence {
            tunnel: w539 -> [w549]
            tunnel: w540 -> [w550]
            tunnel: w541 -> [w551]
            tunnel: w530 -> [w544]
            tunnel: [w544] -> w538
            tunnel: [w551] -> w537
            tunnel: [w550] -> w536
            tunnel: [w548] -> w535
            tunnel: [w547] -> w534
            tunnel: [w545] -> w533
            tunnel: [w543] -> w532
            tunnel: [w549] -> w531
            tunnel: w529 -> [w546]
            tunnel: w538 -> [w562]
            tunnel: w537 -> [w560]
            tunnel: w536 -> [w559]
            tunnel: w535 -> [w557]
            tunnel: w534 -> [w556]
            tunnel: w533 -> [w555]
            tunnel: w532 -> [w554]
            tunnel: w531 -> [w552]
            tunnel: [w561] -> w528
            tunnel: [w558] -> w527
            tunnel: [w553] -> w526
            tunnel: [w608] -> w542
            tunnel: w528 -> [w608]
            tunnel: w527 -> [w607]
            tunnel: w526 -> [w606]
            tunnel: [w607] -> w525
            tunnel: [w606] -> w524
            frame #0 {
              n138 = Unbundle By Name(w544) -> ("Data.Connect"=w548:T1, "Data.Func"=w547:T7)
              n139 = call "MLLF_CommandDelimeter.vi"("command with param"=w546) -> ("command"=w545:string, "Spit delimetre"=w543:string)  [unwired: 6 in, 3 out]
            }
            frame #1 {
              n140 = case shown="\"#\", \"SCPI\"" w555 {
                selector: w555 -> [w564 _ _ _ _ _ _]
                tunnel: [w563 _ w572 w584 _ w588 w600] -> w558
                tunnel: w560 -> [_ _ _ _ _ _ _]
                tunnel: [w565 w566 w581 w585 w586 w597 w605] -> w561
                tunnel: w562 -> [w565 w566 w581 w585 w586 w597 w605]
                tunnel: w557 -> [_ _ w574 _ _ w596 w604]
                tunnel: w559 -> [_ _ _ _ _ _ _]
                tunnel: w554 -> [_ _ w568 _ _ _ _]
                tunnel: w556 -> [_ _ _ _ _ _ _]
                tunnel: [_ _ w573 w582 _ w589 w598] -> w553
                tunnel: w552 -> [_ _ _ w584 _ _ _]
                frame "False", Default {
                  n141 = call "MLLF_UnknownCommand(SubVI).vi"("Unknown command"=w564) -> ("error out"=w563:errorcluster)  [unwired: 10 in]
                }
                frame "______________ Standart ________________" {
                }
                frame "#", "SCPI" {
                  n142 = Search and Replace String(replace all?=TRUE ("replace all? (F)"), input string=w568, search string="''", replace string="\"" ("replace string (\"\")")) -> (result string=w567:string)  [unwired: 4 in, 3 out]
                  n143 = call "MLLF_ClearBuffer.vi"("Timeout(default = 300 ms)"=u32 100 ("Timeout"), "DriverConnect in"=w574) -> ("Error Out"=w575:errorcluster, "DriverConnect out"=w576:T1)  [unwired: 6 in, 1 out]
                  n144 = call "MLLF_WriteToBufferWithDelay.vi"("Delay Time ( 0,05 s)"=0.1 ("Delay Time (s)"), "Command"=w567, "Error In"=w575, "DriverConnect in"=w576) -> ("Error Out"=w579:errorcluster, "DriverConnect out"=w580:T1)  [unwired: 6 in]
                  n145 = call "MLLF_ReadBuffer.vi"("Error In"=w579, "DriverConnect in"=w580) -> ("Error Out"=w572:errorcluster, "String"=w573:string)  [unwired: 6 in, 1 out]
                }
                frame "TIMEOUT" {
                  n146 = Unbundle By Name(w585) -> ("Data.Connect.InterfaceSettings.TMO, ms"=w583:i32)
                  n147 = Format Value(value (0)=w583) -> (output string=w582:string)  [unwired: 2 in]
                }
                frame "________________________________________" {
                }
                frame "READ" {
                  n148 = call "MLLF_WriteToBufferWithDelay.vi"("Delay Time ( 0,05 s)"=0.05 ("Delay Time (s)"), "Command"="READ?" ("String"), "DriverConnect in"=w596) -> ("Error Out"=w595:errorcluster, "DriverConnect out"=w594:T1)  [unwired: 7 in]
                  n149 = call "MLLF_ReadBuffer.vi"("Error In"=w595, "DriverConnect in"=w594) -> ("Error Out"=w588:errorcluster, "String"=w591:string)  [unwired: 6 in, 1 out]
                  n150 = Fract/Exp String To Number(use system decimal point (T)=FALSE, string=w591) -> (number=w590:dbl)  [unwired: 2 in, 1 out]
                  n151 = Format Value(value (0)=w590) -> (output string=w589:string)  [unwired: 2 in]
                }
                frame "FUNC" {
                  n152 = call "MLLF_WriteToBufferWithDelay.vi"("Delay Time ( 0,05 s)"=0.05 ("Delay Time (s)"), "Command"="MEASure:CURRent:AC?" ("String"), "DriverConnect in"=w604) -> ("Error Out"=w603:errorcluster, "DriverConnect out"=w602:T1)  [unwired: 7 in]
                  n153 = call "MLLF_ReadBuffer.vi"("Error In"=w603, "DriverConnect in"=w602) -> ("Error Out"=w600:errorcluster, "String"=w598:string)  [unwired: 6 in, 1 out]
                }
              }
            }
            frame #2 {
            }
          }
        }
        frame "close" {
          n154 = Unbundle By Name(w610) -> ("Data.Connect.OpenedSession"=w612:T3)
          n155 = VISA Close(VISA resource name=w612) -> (error out=w611:errorcluster)  [unwired: 1 in]
        }
      }
    }
    frame Error {
    }
  }
  n156 = local write "Settings"(w1) -> ()
  n157 = flat-sequence {
    tunnel: [w624] -> w2
    tunnel: [w623] -> w4
    tunnel: w7 -> [w622]
    tunnel: w5 -> [w621]
    tunnel: w6 -> [w617]
    tunnel: [w619] -> w3
    frame #0 {
      # "driver out"
      n158 = Unbundle By Name(w617) -> ("Data"=w616:cluster{"Connect":T1, "Channel":T6, "Func":T7})
      n159 = To Variant(anything=w616) -> (Variant=w618:variant)
      n160 = Bundle By Name(cluster=w617, "Saved Data"=w618) -> (w619:T8)
      n161 = call "MLLF_SaveLastSettingUtility.vi"("error in"=w621, "Saved Data"=w618) -> ("error out"=w620:T14)  [unwired: 8 in, 1 out]
      n162 = call "MCF_Output.vi"("Error In"=w620, "Input"=w622) -> ("Error Out"=w623:errorcluster, "Output"=w624:string)  [unwired: 8 in]
    }
  }
  n163 = local write "Settings"(w3) -> ()
  "error out" <- w4
  "Response" <- w2
